vi "Update Screen.vi"(8 "error in (no error)":errorcluster, 11 "Update Screen":T1) -> (0 "error out":errorcluster)   [LabVIEW 2016]
uses:
  Update Screen.ctl
  <vilib>/addons/Display/_Lib/Typedefs/cRIO_Display_Typedefs_DisplayMode.ctl
  <vilib>/addons/Display/_Lib/Typedefs/cRIO_Display_Typedefs_StringConfig.ctl
  <vilib>/addons/Display/_Lib/Typedefs/cRIO_Display_Typedefs_Fonts.ctl
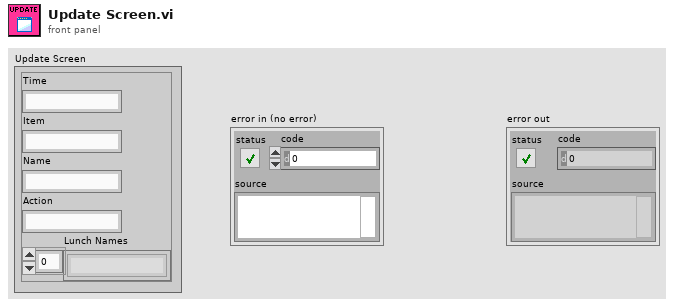
[diagram p1: front panel]
types:
  T1 = typedef "Update Screen.ctl" = cluster{"Time":string, "Item":string, "Name":string, "Action":string, "Lunch Names":string[]}
  T2 = typedef "cRIO_Display_Typedefs_StringConfig.ctl" = cluster{"Column":u8, "Row":u8, "StringColor":u32, "Fontsize":T3}
  T3 = typedef "cRIO_Display_Typedefs_Fonts.ctl" = enum8{"Small", "Medium", "Large", "XLarge"}
  T4 = typedef "cRIO_Display_Typedefs_DisplayMode.ctl" = enum16{"Landscape", "Landscape Rotated", "Portrait", "Portrait Rotated"}
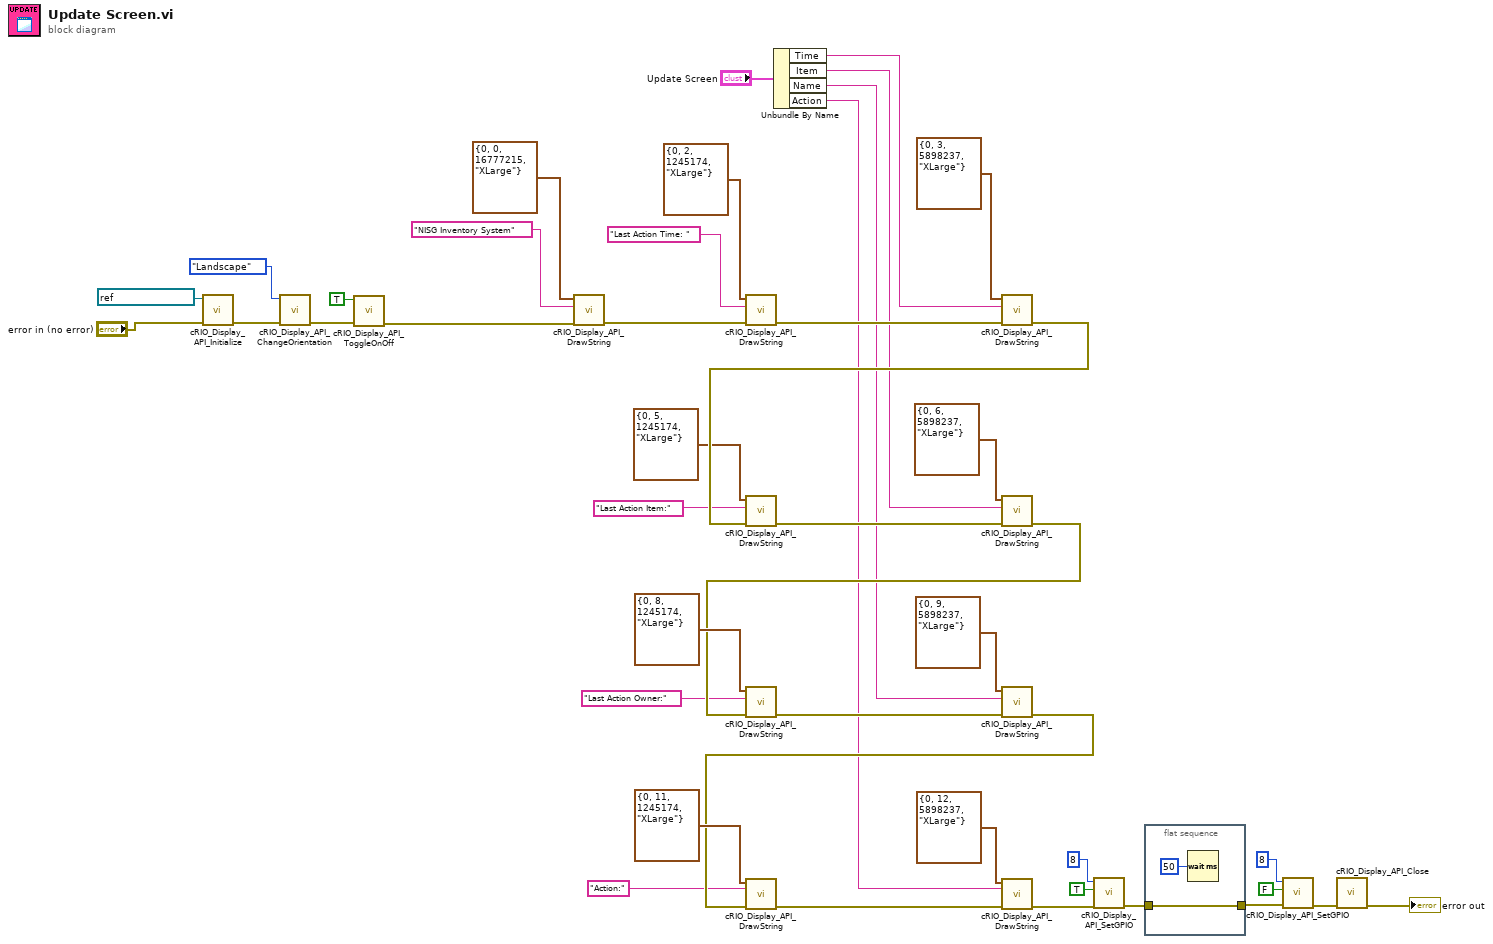
[diagram p0: block diagram]
diagram:
  n1 = call <vilib>:"cRIO_Display_API_Initialize.vi"("error in"="error in (no error)", "cRIODisplay Port"=refnum<visa-resource-name> "ASRL1::INSTR") -> ("error out"=w42:errorcluster)  [unwired: 9 in]
  n2 = call <vilib>:"cRIO_Display_API_ChangeOrientation.vi"("error in"=w42, "DisplayMode"=cRIO_Display_Typedefs_DisplayMode."Landscape") -> ("error out"=w16:errorcluster)  [unwired: 9 in]
  n3 = call <vilib>:"cRIO_Display_API_ToggleOnOff.vi"("error in"=w16, "On/Off"=TRUE) -> ("error out"=w14:errorcluster)  [unwired: 9 in]
  n4 = call <vilib>:"cRIO_Display_API_DrawString.vi"("error in"=w14, "String"="NISG Inventory System", "StringConfig"=T2 {"Column"=0, "Row"=0, "StringColor"=16777215, "Fontsize"=enum."XLarge"}) -> ("error out"=w21:errorcluster)  [unwired: 8 in]
  n5 = call <vilib>:"cRIO_Display_API_DrawString.vi"("error in"=w21, "String"="Last Action Time: ", "StringConfig"=T2 {"Column"=0, "Row"=2, "StringColor"=1245174, "Fontsize"=enum."XLarge"}) -> ("error out"=w39:errorcluster)  [unwired: 8 in]
  n6 = Unbundle By Name("Update Screen") -> ("Time"=w4:string, "Item"=w3:string, "Name"=w2:string, "Action"=w1:string)
  n7 = call <vilib>:"cRIO_Display_API_DrawString.vi"("error in"=w39, "String"=w4, "StringConfig"=T2 {"Column"=0, "Row"=3, "StringColor"=5898237, "Fontsize"=enum."XLarge"}) -> ("error out"=w36:errorcluster)  [unwired: 8 in]
  n8 = call <vilib>:"cRIO_Display_API_DrawString.vi"("error in"=w36, "String"="Last Action Item:", "StringConfig"=T2 {"Column"=0, "Row"=5, "StringColor"=1245174, "Fontsize"=enum."XLarge"}) -> ("error out"=w35:errorcluster)  [unwired: 8 in]
  n9 = call <vilib>:"cRIO_Display_API_DrawString.vi"("error in"=w35, "String"=w3, "StringConfig"=T2 {"Column"=0, "Row"=6, "StringColor"=5898237, "Fontsize"=enum."XLarge"}) -> ("error out"=w26:errorcluster)  [unwired: 8 in]
  n10 = call <vilib>:"cRIO_Display_API_DrawString.vi"("error in"=w26, "String"="Last Action Owner:", "StringConfig"=T2 {"Column"=0, "Row"=8, "StringColor"=1245174, "Fontsize"=enum."XLarge"}) -> ("error out"=w34:errorcluster)  [unwired: 8 in]
  n11 = call <vilib>:"cRIO_Display_API_DrawString.vi"("error in"=w34, "String"=w2, "StringConfig"=T2 {"Column"=0, "Row"=9, "StringColor"=5898237, "Fontsize"=enum."XLarge"}) -> ("error out"=w25:errorcluster)  [unwired: 8 in]
  n12 = call <vilib>:"cRIO_Display_API_DrawString.vi"("error in"=w25, "String"="Action:", "StringConfig"=T2 {"Column"=0, "Row"=11, "StringColor"=1245174, "Fontsize"=enum."XLarge"}) -> ("error out"=w33:errorcluster)  [unwired: 8 in]
  n13 = call <vilib>:"cRIO_Display_API_DrawString.vi"("error in"=w33, "String"=w1, "StringConfig"=T2 {"Column"=0, "Row"=12, "StringColor"=5898237, "Fontsize"=enum."XLarge"}) -> ("error out"=w13:errorcluster)  [unwired: 8 in]
  n14 = call <vilib>:"cRIO_Display_API_SetGPIO.vi"("error in"=w13, "GPIO State"=TRUE, "GPIO Pin"=u8 8) -> ("error out"=w8:errorcluster)  [unwired: 8 in]
  n15 = flat-sequence {
    tunnel: w8 -> [w44]
    tunnel: [w44] -> w7
    frame #0 {
      n16 = Wait (ms)(milliseconds to wait=u32 50) -> ()  [unwired: 1 out]
    }
  }
  n17 = call <vilib>:"cRIO_Display_API_SetGPIO.vi"("error in"=w7, "GPIO State"=FALSE, "GPIO Pin"=u8 8) -> ("error out"=w6:errorcluster)  [unwired: 8 in]
  n18 = call <vilib>:"cRIO_Display_API_Close.vi"("error in"=w6) -> ("error out"=→"error out":errorcluster)  [unwired: 10 in]
